vi "Delete Template VIs.vi"(11 "LVClass":refnum<vi>) -> (3 "LVClass Dup":refnum<vi>)   [LabVIEW 2013]
doc: "Copyright (c) 2016 Sze Howe Koh\n\nThis Source Code Form is subject to the terms of the Mozilla Public License, v. 2.0. If a copy of the MPL was not distributed with this file, You can obtain one at http://mozilla.org/MPL/2.0/."
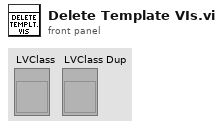
[diagram p1: front panel]
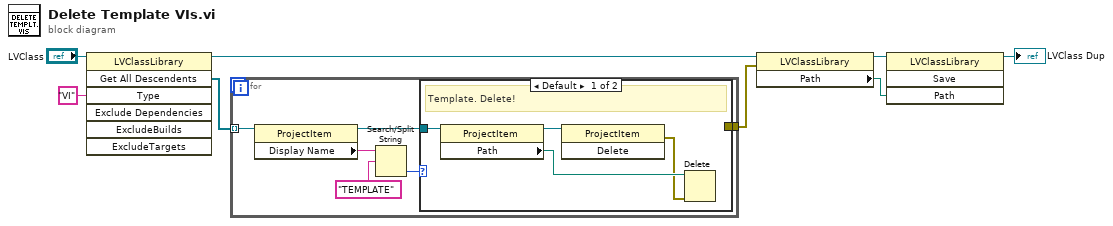
[diagram p0: block diagram]
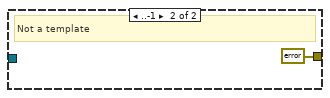
[diagram p2: hidden frame]
diagram:
  n1 = invoke class="LVClassLibrary" method="Get All Descendents"(reference="LVClass", "Type"="VI") -> (reference out=w5:refnum<vi>, "All Descendents"=w6:refnum<vi>[])  [unwired: 5 in, 5 out]
  n2 = for {
    tunnel: w6 -> [w14] mode=indexing
    tunnel: [w9] -> w2
    n3 = property class="ProjectItem"(reference=w14) -> (reference out=w10:refnum<vi>, "Display Name"=w13:string)  [unwired: 1 in, 1 out]
    n4 = Search/Split String(string=w13, search string/char (-)="TEMPLATE") -> (offset of match=w11:i32)  [unwired: 1 in, 2 out]
    n5 = case shown="Default" w11 {
      tunnel: w10 -> [w18 _]
      tunnel: [_ errorcluster {"status"=FALSE, "code"=0, "source"=""} ("error out")] -> w9
      frame Default {
        # "Template. Delete!"
        n6 = property class="ProjectItem"(reference=w18) -> (reference out=w17:refnum<vi>, "Path"=w16:path)  [unwired: 1 in, 1 out]
        n7 = invoke class="ProjectItem" method="Delete"(reference=w17) -> (error out=w15:errorcluster)  [unwired: 2 in, 2 out]
        n8 = Delete(path (use dialog)=w16, error in=w15) -> ()  [unwired: 3 in, 3 out]
      }
      frame ..-1 {
        # "Not a template"
      }
    }
  }
  n9 = property class="LVClassLibrary"(reference=w5, error in=w2) -> (reference out=w4:refnum<vi>, "Path"=w3:path)  [unwired: 1 out]
  n10 = invoke class="LVClassLibrary" method="Save"(reference=w4, "Path"=w3) -> (reference out=→"LVClass Dup":refnum<vi>)  [unwired: 2 in, 3 out]
